vi "RSNRPZ Initialize.vi"(8 "error in (no error)":errorcluster, 9 "Reset Device (T:Reset Device)":bool=TRUE, 10 "ID Query (T:Do Query)":bool=TRUE, 11 "Resource Name (USB::0x0aad::0x000b::100000)":string="USB::0x0aad::0x000b::100000") -> (0 "error out":errorcluster, 3 "dup VISA session":refnum<visa-resource-name>)   [LabVIEW 2014]
doc: "This VI performs the following initialization actions and assigned specified sesnor to channel 1:\n\n- Opens a session to the specified device using the interface and address specified in the Resource Name control.\n\n- Performs an identification query on the sensor.\n\n- Resets the instrument to a known state.\n\n- Sends initialization commands to the sensor\n\n- Returns an Instrument Handle which is used to differentiate between different sessions of this instrument driver.\n\nNote:\n\n1) Do not initilize every sensor with RSNRPZ Initialize.vi. if you want comunicate with more sensor use RSNRPZ Add Sensor.vi for adding a new channel. The reason is the RSNRPZ Close.vi destroys all sensor sessions assigned to process."
uses:
  rsnrpz_32.dll
panel:
  # "Warning: The driver requires NRP Toolkit installed on your computer"
  # "Don't initialize 2 sensors with init function. Use Add Sensor and read function help."
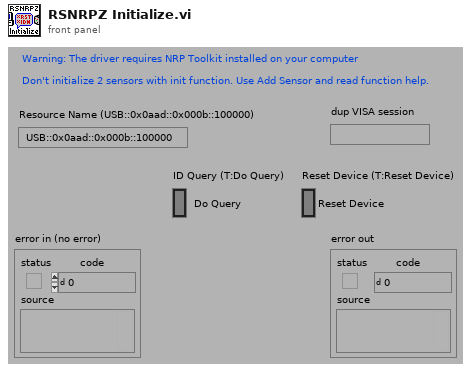
[diagram p1: front panel]
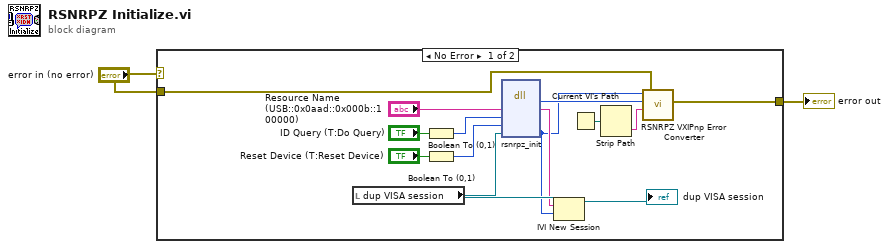
[diagram p0: block diagram]
diagram:
  n1 = case shown="No Error" "error in (no error)" {
    tunnel: "error in (no error)" -> [w7 w17]
    tunnel: [w8 w17] -> w1
    frame No Error {
      n2 = local read "dup VISA session"() -> (w12:refnum<visa-resource-name>)
      n3 = Boolean To (0,1)(Boolean="ID Query (T:Do Query)") -> (0, 1=w4:i16)
      n4 = Boolean To (0,1)(Boolean="Reset Device (T:Reset Device)") -> (0, 1=w13:i16)
      n5 = dll-call lib="rsnrpz_32.dll" fn="rsnrpz_init"("resourceName"="Resource Name (USB::0x0aad::0x000b::100000)", "IDQuery"=w4, "resetDevice"=w13, "instrumentHandle"=w12) -> (w14:i32, "resourceName"=w11:string, "instrumentHandle"=w10:i32)  [unwired: 5 in, 2 out]
      n6 = IVI New Session(9:w10, 10:w11, 11:w12) -> (3:→"dup VISA session":refnum<visa-resource-name>)
      n7 = Current VI's Path() -> (path=w6:path)
      n8 = Strip Path(path=w6) -> (name=w5:string)  [unwired: 1 out]
      n9 = call "RSNRPZ VXIPnp Error Converter.vi"("error in (no error)"=w7, "name of VI"=w5, "VXIPnp error code"=w14, "VISA session"=w10) -> ("error out"=w8:errorcluster)  [unwired: 1 out]
    }
    frame Error {
    }
  }
  "error out" <- w1
